vi "Design Engine.vi"() -> ()   [LabVIEW 2012, in "Design Server.lvlib"]
uses:
  Design Server.lvlib
  Design Request.ctl
  Variable cluster.ctl
  Method.ctl
  ReadWrite.ctl
panel:
  in  "Open Helper Apps":bool=TRUE
  in  "Pause":bool=TRUE
  in  "File Directories":bool
  out "stop loops":bool
  in  "stop":bool
  in  "Tab Control":T1(tab)=enum."Version Control"
  out "Find-Replace":cluster{"Find":string, "Replace":string}[](array[cluster])
  out "DesignRequest":T2
  out "Mathcad Output":T3
  out "Pending Client":i32
  out "progress":cluster{"Progress":u8, "AC variable":string} {"Progress" scale=0.0..100.0}
  out "Pending Stock":i16
  out "Current Revision":i32
  in  "Method Version":i32 min=0 max=7195
  in  "Methods":u16(ring) items=["EtFlocSedFi", "EtFlocSedFiHigh", "Flocculator", "SedTank", "LFOM", "SRSF", "PAClCdc", "Cdc", "Box", "EtFlocSedFiLow", "EntTank"]
  out "Method Description":T4
  out "Method Version":i32
  out "init errors":errorcluster caption="error out"
  out "design errors":errorcluster
  out "Successful Checkout":bool
  out "Load CAD":errorcluster
  out "Web address":string
  in  "millisecond loop delay":u32=5000
  out "Loaded CAD":bool
  # "The method version sets the version used for all method files. A zero means use the current version.\n\nGiven a method version from the master method file, SVN checkout is used to load that version of the Mathcad source files."
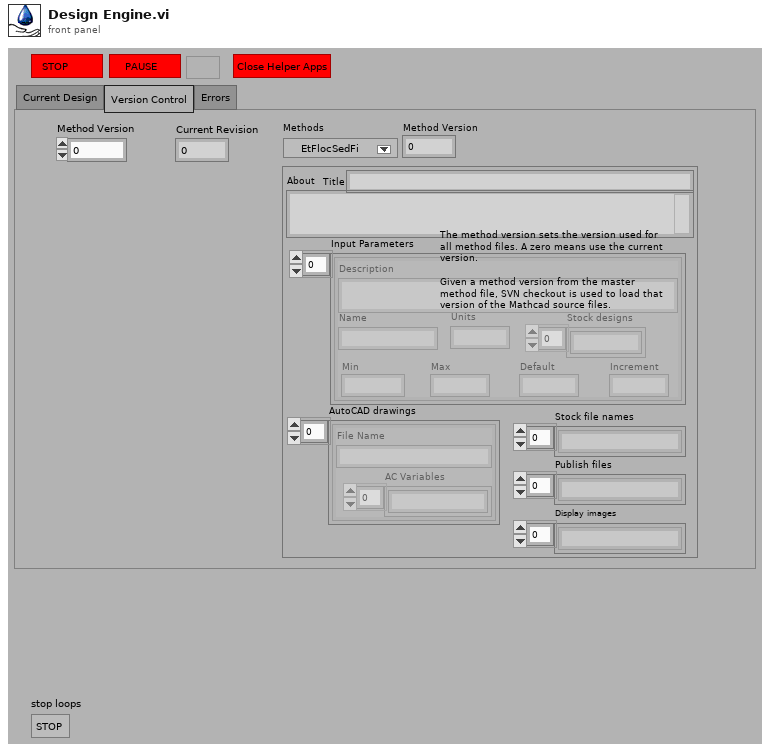
[diagram p1: front panel]
types:
  T1 = enum32{"Current Design", "Version Control", "Errors"}
  T2 = typedef "Design Server.lvlib/Design Request.ctl" = cluster{"Project Folder":path, "Method Name":string, "Inputs":T3, "Version":i32}
  T3 = typedef "Design Server.lvlib/Variable cluster.ctl" = cluster{"Label.Text":string, "Control Type":u32, "Numeric":dbl, "Array":dbl[], "status":bool, "Str Array":string[], "String":string, "unit":string}[]
  T4 = typedef "Method.ctl" = cluster{"Title":string, "About":string, "Input Parameters":cluster{"Description":string, "Name":string, "Min":string, "Max":string, "Default":string, "Units":string, "Increment":string, "Stock designs":string[]}[], "AutoCAD drawings":cluster{"File Name":string, "AC Variables":string[]}[], "Stock file names":string[], "Publish files":string[], "Display images":string[]}
  T5 = typedef "ReadWrite.ctl" = enum16{"Read", "Write"}
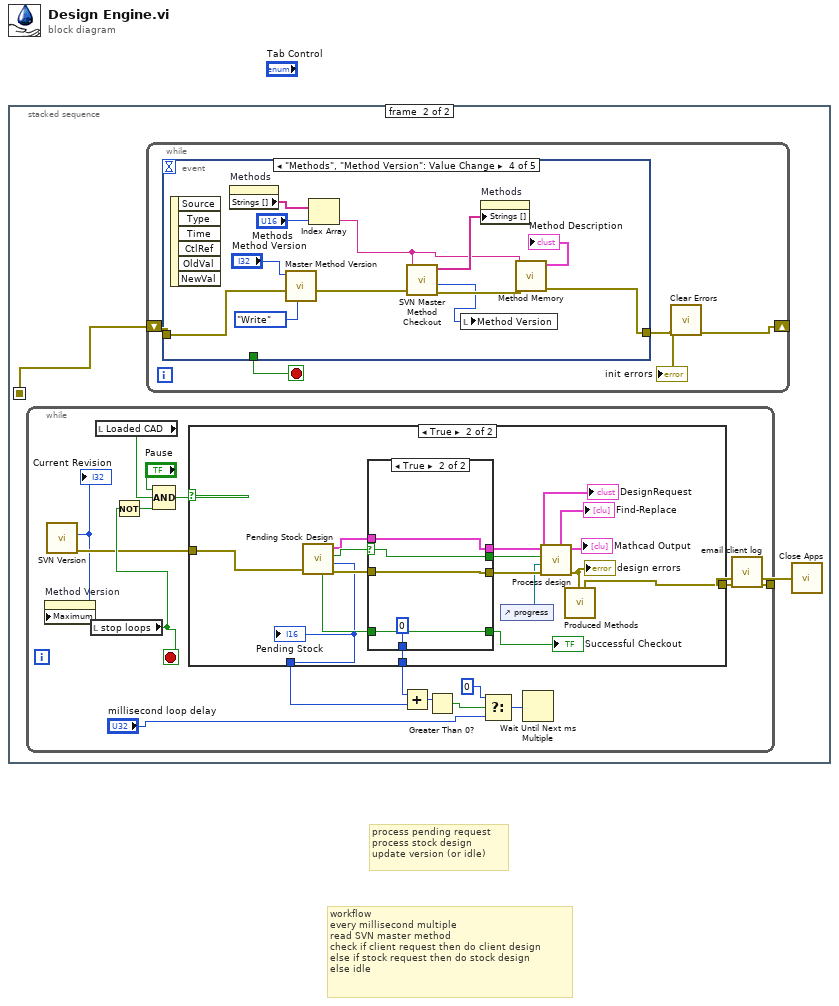
[diagram p0: block diagram]
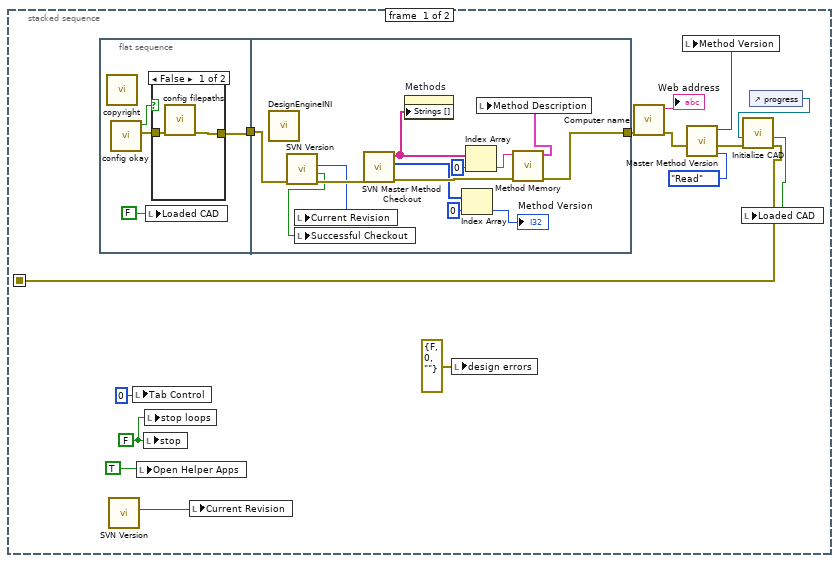
[diagram p2: hidden frame]
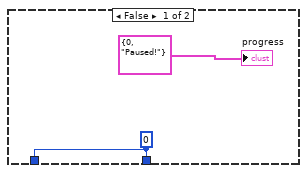
[diagram p4: hidden frame]
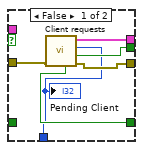
[diagram p5: hidden frame]
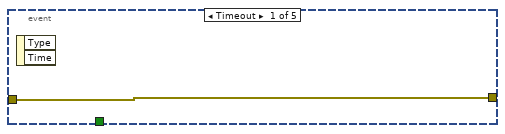
[diagram p6: hidden frame]
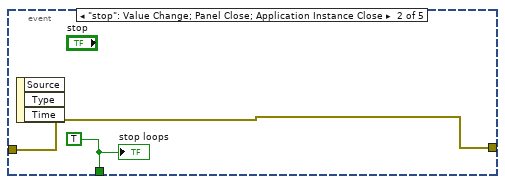
[diagram p7: hidden frame]
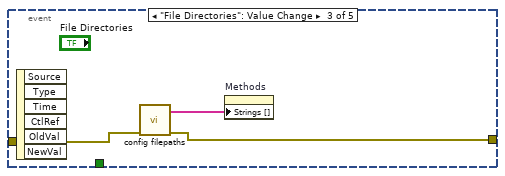
[diagram p8: hidden frame]
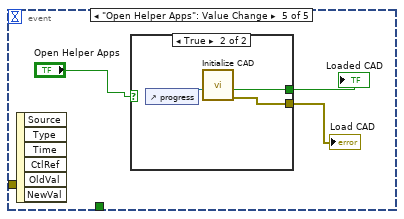
[diagram p9: hidden frame]
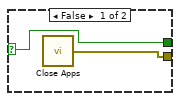
[diagram p10: hidden frame]
diagram:
  # "workflow\nevery millisecond multiple\nread SVN master method\ncheck if client request then do client design\nelse if stock request then do stock design\nelse idle"
  # "process pending request\nprocess stock design\nupdate version (or idle)"
  n1 = stacked-sequence {
    seq-local: [w3 _] -> [_ w37]
    frame #0 {
      w7 = FALSE ("stop")
      n2 = flat-sequence {
        tunnel: [w19] -> w13
        tunnel: [w34] -> w14
        tunnel: w13 -> [w26]
        frame #0 {
          n3 = call "copyright.vi"() -> ()  [unwired: 4 in]
          n4 = call "config okay.vi"() -> ("error out"=w16:errorcluster, "config okay"=w17:bool)  [unwired: 10 in]
          n5 = local write "Loaded CAD"(FALSE ("Loaded CAD")) -> ()
          n6 = case shown="False" w17 {
            tunnel: [w21 w22] -> w19
            tunnel: w16 -> [w20 w22]
            frame False {
              n7 = call "config filepaths.vi"("error in (no error)"=w20) -> ("error out"=w21:errorcluster)  [unwired: 9 in, 1 out]
            }
            frame True {
            }
          }
        }
        frame #1 {
          n8 = call "DesignEngineINI.vi"() -> ()  [unwired: 6 in, 2 out]
          n9 = call "SVN Version.vi"("error in (no error)"=w26) -> ("error out"=w25:errorcluster, "Successful version check"=w23:bool, "Revision"=w24:i32)  [unwired: 7 in, 1 out]
          n10 = local write "Current Revision"(w24) -> ()
          n11 = local write "Successful Checkout"(w23) -> ()
          n12 = call "SVN Master Method Checkout.vi"("error in (no error)"=w25) -> ("error out"=w35:errorcluster, "versions"=w30:i32[], "Method Names"=w27:string[])  [unwired: 5 in, 3 out]
          n13 = property on="Methods" class="Ring (strict)"("Strings []"=w27) -> ()  [unwired: 2 in, 2 out]
          n14 = Index Array(array=w30, index=0) -> (element=→"Method Version":i32)
          n15 = Index Array(array=w27, index=0) -> (element=w32:string)
          n16 = call "Method Memory.vi"("error in"=w35, "Method Name"=w32) -> ("error out"=w34:errorcluster, "Method Out"=w28:T4)  [unwired: 7 in, 1 out]
          n17 = local write "Method Description"(w28) -> ()
        }
      }
      n18 = call "SVN Version.vi"() -> ("Revision"=w10:i32)  [unwired: 8 in, 3 out]
      n19 = local write "Tab Control"(u8 0 ("Disabled")) -> ()
      n20 = local write "Open Helper Apps"(TRUE ("Open Helper Apps")) -> ()
      n21 = local write "stop"(w7) -> ()
      n22 = local write "stop loops"(w7) -> ()
      n23 = local write "Current Revision"(w10) -> ()
      n24 = local write "design errors"(errorcluster {"status"=FALSE, "code"=0, "source"=""} ("design errors")) -> ()
      n25 = call "Computer name.vi"("error in (no error)"=w14) -> ("error out"=w6:errorcluster, "Computer web address"=→"Web address":string)  [unwired: 8 in, 1 out]
      n26 = call "Master Method Version.vi"("Config"=ReadWrite."Read", "error in (no error)"=w6) -> ("error out"=w4:errorcluster, "Master Method Version"=w8:i32)  [unwired: 6 in, 2 out]
      n27 = local write "Method Version"(w8) -> ()
      n28 = control-ref of="progress"() -> (w2:refnum<vi>)
      n29 = call "Initialize CAD.vi"("error in (no error)"=w4, "progress"=w2) -> ("error out"=w3:errorcluster, "Success"=w1:bool)  [unwired: 8 in]
      n30 = local write "Loaded CAD"(w1) -> ()
    }
    frame #1 {
      n31 = while {
        tunnel: [w38] -> w36
        stop <- w50 stop-if-true
        n32 = call "SVN Version.vi"() -> ("error out"=w41:errorcluster, "Revision"=w40:i32)  [unwired: 8 in, 2 out]
        "Current Revision" <- w40
        n33 = property on="Method Version" class="DigNum (strict)"("Maximum"=w40) -> ()  [unwired: 2 in, 2 out]
        n34 = local read "stop loops"() -> (w50:bool)
        n35 = local read "Loaded CAD"() -> (w52:bool)
        n36 = Not(x=w50) -> (.not. x?=w51:bool)
        n37 = Compound Arithmetic op=AND("Pause", w52, w51) -> (w49:bool)
        n38 = case shown="True" w49 {
          tunnel: [_ w71] -> w39
          tunnel: [w54 w58] -> w48
          tunnel: [w54 w57] -> w47
          tunnel: w41 -> [_ w56]
          frame False {
            w54 = 0 ("Number of Pending Requests")
            "progress" <- cluster{"Progress":u8, "AC variable":string} {"Progress"=0, "AC variable"="Paused!"} ("progress")
          }
          frame True {
            n39 = call "Pending Stock Design.vi"("error in (no error)"=w56) -> ("error out"=w61:errorcluster, "Pending"=w58:i16, "Need a design"=w63:bool, "DesignRequest"=w62:T2, "Successful Checkout"=w59:bool)  [unwired: 5 in, 1 out]
            "Pending Stock" <- w58
            n40 = case shown="True" w63 {
              selector: w63 -> [_ w81]
              tunnel: [w75 w80] -> w70
              tunnel: [w74 w81] -> w69
              tunnel: [w77 w82] -> w68
              tunnel: w62 -> [_ w82]
              tunnel: w61 -> [w76 w80]
              tunnel: [w73 w79] -> w60
              tunnel: w59 -> [_ w79]
              tunnel: [w72 0 ("Number of Pending Requests")] -> w57
              frame False {
                n41 = call "Client requests.vi"("error in"=w76) -> ("error out"=w75:errorcluster, "Good request"=w74:bool, "Number of Pending Requests"=w72:i32, "DesignRequest"=w77:T2, "Successful Checkout"=w73:bool)  [unwired: 6 in]
                "Pending Client" <- w72
              }
              frame True {
              }
            }
            "DesignRequest" <- w68
            "Successful Checkout" <- w60
            n42 = control-ref of="progress"() -> (w65:refnum<vi>)
            n43 = call "Process design.vi"("error in (no error)"=w70, "progress"=w65, "Request Pending"=w69, "DesignRequest"=w68) -> ("design error"=w64:errorcluster, "Mathcad Output"=→"Mathcad Output":T3, "Find-Replace"=→"Find-Replace":cluster{"Find":string, "Replace":string}[])  [unwired: 3 in, 2 out]
            "design errors" <- w64
            n44 = call "Produced Methods.vi"("error in"=w64) -> ("error out"=w71:errorcluster)  [unwired: 9 in, 1 out]
          }
        }
        n45 = Add(x=w47, y=w48) -> (x+y=w46:i32)
        n46 = Greater Than 0?(x=w46) -> (x > 0?=w45:bool)
        n47 = Select(t=0 ("Number of Pending Requests"), s=w45, f="millisecond loop delay") -> (s? t:f=w42:u32)
        n48 = Wait Until Next ms Multiple(millisecond multiple=w42) -> ()  [unwired: 1 out]
        n49 = call "email client log.vi"("error in"=w39) -> ("error out"=w38:errorcluster)  [unwired: 10 in]
      }
      n50 = while {
        shift-right: [w83] -> _
        shift-left: w37 -> [w85]
        stop <- w86 stop-if-true
        n51 = event shown="[3] \"Methods\", \"Method Version\": Value Change" {
          selector: _ -> [_ _ _ _ _]
          dyn-events: _ -> [_ _ _ _ _]
          timeout: _ -> [_ _ _ _ _]
          tunnel: [_ w89 _ _ _] -> w86
          tunnel: [w87 w88 w92 w104 _] -> w84
          tunnel: w85 -> [w87 w88 w91 w93 _]
          event Timeout {
            n52 = event-data() -> ()  [unwired: 1 in, 2 out]
          }
          event "stop": Value Change; Panel Close; Application Instance Close {
            w89 = TRUE
            n53 = event-data() -> ()  [unwired: 1 in, 3 out]
            "stop loops" <- w89
          }
          event "File Directories": Value Change {
            n54 = event-data() -> ()  [unwired: 1 in, 6 out]
            n55 = call "config filepaths.vi"("error in (no error)"=w91) -> ("error out"=w92:errorcluster, "Methods"=w90:string[])  [unwired: 9 in]
            n56 = property on="Methods" class="Ring (strict)"("Strings []"=w90) -> ()  [unwired: 2 in, 2 out]
          }
          event "Methods", "Method Version": Value Change {
            n57 = event-data() -> ()  [unwired: 1 in, 6 out]
            n58 = property on="Methods" class="Ring (strict)"() -> ("Strings []"=w102:string[])  [unwired: 2 in, 2 out]
            n59 = call "Master Method Version.vi"("Config"=ReadWrite."Write", "error in (no error)"=w93, "Master Method version"="Method Version") -> ("error out"=w94:errorcluster)  [unwired: 5 in, 3 out]
            n60 = Index Array(array=w102, index="Methods") -> (element=w97:string)
            n61 = call "SVN Master Method Checkout.vi"("error in (no error)"=w94, "Method Name"=w97) -> ("error out"=w99:errorcluster, "Method Version"=w95:i32, "Method Names"=w100:string[])  [unwired: 4 in, 3 out]
            n62 = local write "Method Version"(w95) -> ()
            n63 = property on="Methods" class="Ring (strict)"("Strings []"=w100) -> ()  [unwired: 2 in, 2 out]
            n64 = call "Method Memory.vi"("error in"=w99, "Method Name"=w97) -> ("error out"=w104:errorcluster, "Method Out"=→"Method Description":T4)  [unwired: 7 in, 1 out]
          }
          event "Open Helper Apps": Value Change {
            n65 = event-data() -> ()  [unwired: 1 in, 6 out]
            n66 = case shown="True" "Open Helper Apps" {
              selector: "Open Helper Apps" -> [w108 _]
              tunnel: [w108 w111] -> w107
              tunnel: [w109 w110] -> w106
              frame False {
                n67 = call "Close Apps.vi"() -> ("error out"=w109:errorcluster)  [unwired: 1 in]
              }
              frame True {
                n68 = control-ref of="progress"() -> (w112:refnum<vi>)
                n69 = call "Initialize CAD.vi"("progress"=w112) -> ("error out"=w110:errorcluster, "Success"=w111:bool)  [unwired: 9 in]
              }
            }
            "Loaded CAD" <- w107
            "Load CAD" <- w106
          }
        }
        "init errors" <- w84
        n70 = call <vilib>:"Clear Errors.vi"("error in (no error)"=w84) -> ("error out"=w83:errorcluster)  [unwired: 6 in]
      }
      n71 = call "Close Apps.vi"("error in"=w36) -> ()  [unwired: 1 out]
    }
  }
